vi "Launch Loggers.vi"(8 "error in (no error)":errorcluster, 11 "Historian Logger in":refnum<class "Historian Logger.lvclass">) -> (0 "error out":errorcluster, 3 "Historian Logger out":refnum<class "Historian Logger.lvclass">)   [LabVIEW 2020, in "VolatusHistorian.lvlib" / "Historian Logger.lvclass"]
uses:
  Historian Logger.lvclass
  C:/dev/lv20CE/relink/lv-volatus/Volatus/Module/Module.lvclass
  Volatus/Module/Module.lvclass/Module.ctl
  Historian Logger.lvclass/Historian Logger.ctl
  Volatus/Module/Module.lvclass
  Volatus/VolatusAPI/VolatusAPI.lvclass
  lv-cdm/CDM-Config/CDM-Config.lvlib
  lv-cdm/CDM-Config/Format.ctl
  lv-cdm/CDM-Config/Precision.ctl
  lv-cdm/CDM-Config/Timezone.ctl
  lv-cdm/CDM-Config/ISO8601 Config.ctl
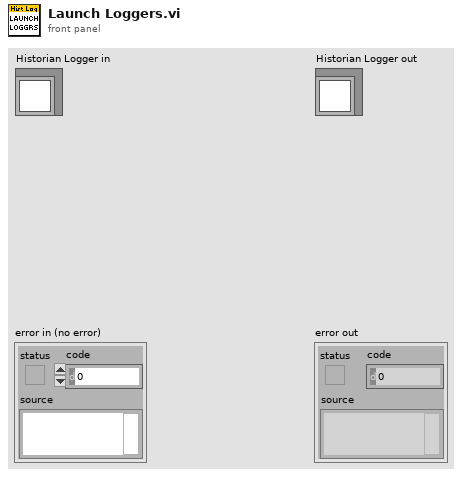
[diagram p1: front panel]
types:
  T1 = typedef "CDM-Config.lvlib/ISO8601 Config.ctl" = cluster{"Format":T2, "Precision":T3, "Timezone":T4}
  T2 = typedef "CDM-Config.lvlib/Format.ctl" = enum16{"Extended", "Basic"}
  T3 = typedef "CDM-Config.lvlib/Precision.ctl" = enum16{"Millisecond", "Second", "Minute", "Hour", "Day"}
  T4 = typedef "CDM-Config.lvlib/Timezone.ctl" = enum16{"UTC", "Local"}
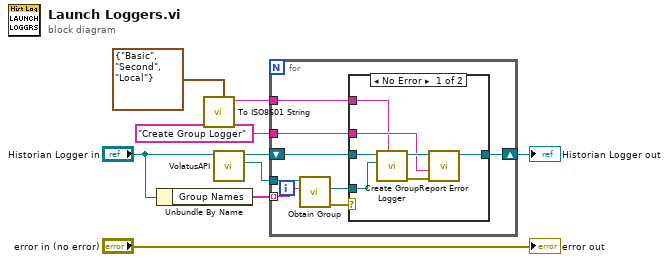
[diagram p0: block diagram]
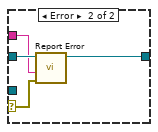
[diagram p2: hidden frame]
diagram:
  n1 = Unbundle By Name("Historian Logger in") -> ("Group Names"=w6:string[])
  n2 = call "To ISO8601 String.vi"("Format Config"=T1 {"Format"=enum."Basic", "Precision"=enum."Second", "Timezone"=enum."Local"}) -> ("ISO 8601"=w1:string)  [unwired: 10 in]
  n3 = call "VolatusAPI.vi"("Module in"="Historian Logger in") -> ("VolatusAPI"=w8:refnum<class "VolatusAPI.lvclass">, "Module out"=w5:refnum<class "Historian Logger.lvclass">)  [unwired: 9 in]
  n4 = for {
    tunnel: w8 -> [w17]
    tunnel: w6 -> [w16] mode=indexing
    shift-right: [w14] -> w3
    shift-left: w5 -> [w15]
    tunnel: "Create Group Logger" -> [w11]
    tunnel: w1 -> [w10]
    n5 = call "Obtain Group.vi"("Group Name"=w16, "VolatusAPI in"=w17) -> ("error out"=w13:errorcluster, "Group"=w12:refnum<class "Group.lvclass">)  [unwired: 7 in, 1 out]
    n6 = case shown="No Error" w13 {
      selector: w13 -> [_ w27]
      tunnel: w15 -> [w24 w28]
      tunnel: [w21 w26] -> w14
      tunnel: w12 -> [w22 _]
      tunnel: w11 -> [w19 w25]
      tunnel: w10 -> [w18 _]
      frame No Error {
        n7 = call "Create Group Logger.vi"("Timestamp"=w18, "Group"=w22, "Historian Logger in"=w24) -> ("error out"=w20:errorcluster, "Historian Logger out"=w23:refnum<class "Historian Logger.lvclass">)  [unwired: 7 in]
        n8 = call "Report Error.vi"("error in (no error)"=w20, "Message (None)"=w19, "Module in"=w23) -> ("Module out"=w21:refnum<class "Historian Logger.lvclass">)  [unwired: 7 in, 1 out]
      }
      frame Error {
        n9 = call "Report Error.vi"("error in (no error)"=w27, "Message (None)"=w25, "Module in"=w28) -> ("Module out"=w26:refnum<class "Historian Logger.lvclass">)  [unwired: 7 in, 1 out]
      }
    }
  }
  "Historian Logger out" <- w3
  "error out" <- "error in (no error)"
